vi "GetSingleton.vi"(10 "Destructor (F)":bool, 11 "Creator (F)":bool) -> (2 "Users":i32, 3 "DataStore":refnum<data-value>)   [LabVIEW 2013, in "SMOConfig.lvlib" / "ConfigManager.Cache.lvclass"]
uses:
  ConfigManager.Cache.lvclass
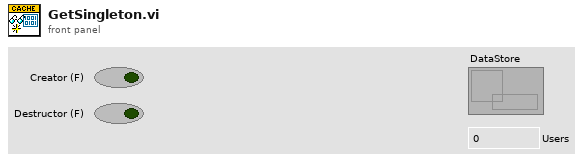
[diagram p1: front panel]
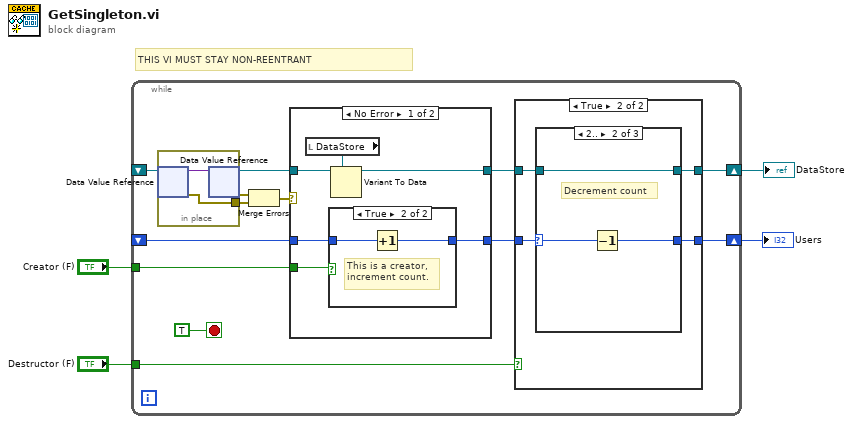
[diagram p0: block diagram]
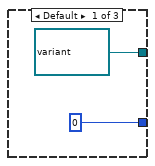
[diagram p3: hidden frame]
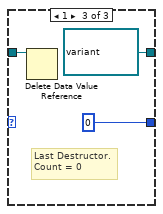
[diagram p4: hidden frame]
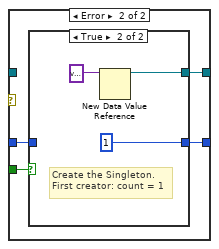
[diagram p6: hidden frame]
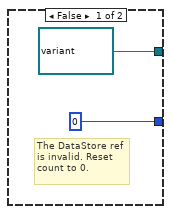
[diagram p7: hidden frame]
diagram:
  # "THIS VI MUST STAY NON-REENTRANT"
  n1 = while {
    shift-right: [w6] -> w2
    shift-left: _ -> [w15]
    tunnel: "Creator (F)" -> [w11]
    shift-right: [w7] -> w1
    shift-left: _ -> [w10]
    tunnel: "Destructor (F)" -> [w5]
    stop <- TRUE stop-if-true
    n2 = in-place {
      in-place-border: [w50] -> w16
      n3 = in-place-dvr #1(w15) -> (w51:variant, w50:errorcluster)
      n4 = in-place-dvr #1(w51) -> (w13:refnum<data-value>, w14:errorcluster)
    }
    n5 = Merge Errors(w14, w16) -> (w12:errorcluster)
    n6 = case shown="No Error" w12 {
      tunnel: [w32 w44] -> w9
      tunnel: w13 -> [w33 _]
      tunnel: w11 -> [w37 w43]
      tunnel: [w35 w42] -> w8
      tunnel: w10 -> [w36 w41]
      frame No Error {
        n7 = local read "DataStore"() -> (w34:refnum<data-value>)
        n8 = case shown="True" w37 {
          tunnel: w36 -> [w38 w40]
          tunnel: [w38 w39] -> w35
          frame False {
            # "Nothing to do.\nRef is valid and\nnot creator."
          }
          frame True {
            # "This is a creator,\nincrement count."
            n9 = Increment(x=w40) -> (x+1=w39:i32)
          }
        }
        n10 = Variant To Data(type=w34, Variant=w33) -> (data=w32:refnum<data-value>)  [unwired: 1 in, 1 out]
      }
      frame Error {
        n11 = case shown="True" w43 {
          tunnel: [refnum<data-value> refnum ("data value reference") w48] -> w44
          tunnel: [0 1] -> w42
          tunnel: w41 -> [_ _]
          frame False {
            # "The DataStore ref\nis invalid. Reset\ncount to 0."
          }
          frame True {
            # "Create the Singleton.\nFirst creator: count = 1"
            n12 = New Data Value Reference(data value=variant ("variant")) -> (data value reference=w48:refnum<data-value>)  [unwired: 1 in, 1 out]
          }
        }
      }
    }
    n13 = case shown="True" w5 {
      tunnel: w9 -> [w19 w21]
      tunnel: [w19 w22] -> w6
      tunnel: w8 -> [w18 w23]
      tunnel: [w18 w20] -> w7
      frame False {
      }
      frame True {
        n14 = case shown="2.." w23 {
          selector: w23 -> [_ w27 _]
          tunnel: [refnum<data-value> refnum ("data value reference") w28 refnum<data-value> refnum ("data value reference")] -> w22
          tunnel: w21 -> [_ w28 w31]
          tunnel: [0 ("Numeric") w26 0 ("Numeric")] -> w20
          frame Default {
          }
          frame 2.. {
            # "Decrement count"
            n15 = Decrement(x=w27) -> (x-1=w26:i32)
          }
          frame 1 {
            # "Last Destructor.\nCount = 0"
            n16 = Delete Data Value Reference(data value reference=w31) -> ()  [unwired: 1 in, 2 out]
          }
        }
      }
    }
  }
  "DataStore" <- w2
  "Users" <- w1
